vi "Load_vs_Position_Simulation_Model.vi"(0 "Load Setpoint":dbl=20.0 format="%#_13g", 7 "Disturbance":dbl=1.0 format="%#_13g") -> (6 "Simulated Load":dbl, 10 "Simulated Position":dbl)   [LabVIEW 2019]
uses:
  <vilib>/Analysis/1siggen.llb/Ramp Pattern by Samples.vi
  <vilib>/Analysis/NI_AALBase.lvlib
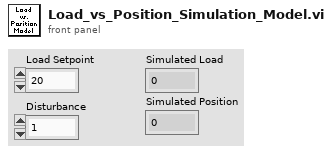
[diagram p1: front panel]
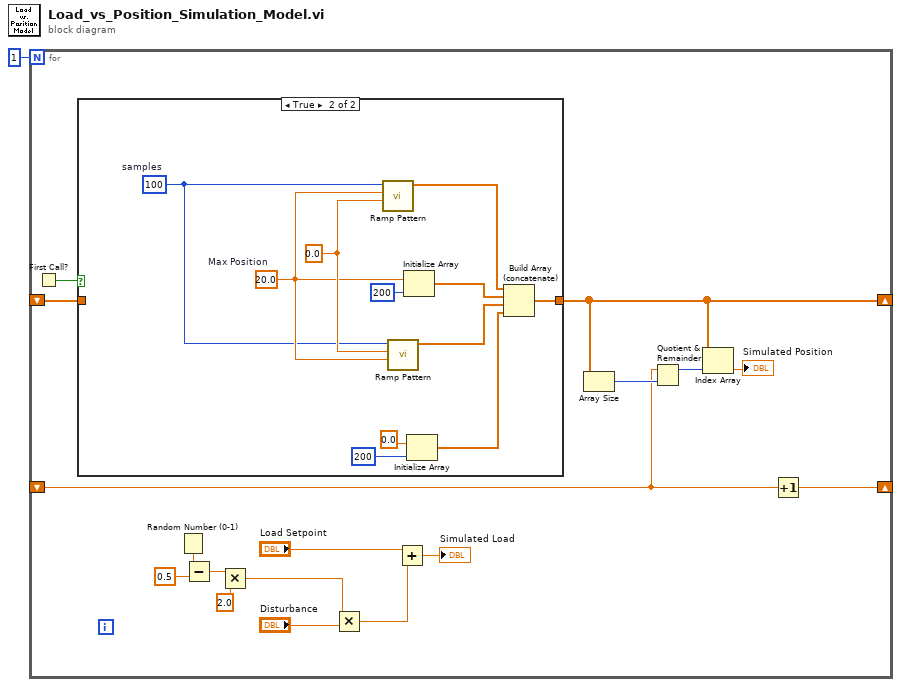
[diagram p0: block diagram]
diagram:
  n1 = for {
    N: 1 -> [_]
    shift-right: [w11] -> _
    shift-left: _ -> [w10]
    shift-right: [w8] -> _
    shift-left: _ -> [w7]
    n2 = First Call?() -> (First Call?: T/F=w9:bool)
    n3 = case shown="True" w9 {
      tunnel: [w19 w30] -> w8
      tunnel: w7 -> [w19 _]
      frame False {
      }
      frame True {
        w21 = 20.0  # Max Position
        w20 = 100  # samples
        w22 = 0.0 ("end")
        n4 = call-poly <vilib>:"Ramp Pattern.vi"("start"=w22, "end"=w21, "samples"=w20) -> ("Ramp Pattern"=w23:dbl[])  [unwired: 7 in, 1 out]
        n5 = call-poly <vilib>:"Ramp Pattern.vi"("start"=w21, "end"=w22, "samples"=w20) -> ("Ramp Pattern"=w25:dbl[])  [unwired: 7 in, 1 out]
        n6 = Initialize Array(w21, 200 ("dimension size")) -> (w26:dbl[])
        n7 = Initialize Array(0.0 ("element"), 200 ("dimension size")) -> (w24:dbl[])
        n8 = Build Array (concatenate)(w23, w26, w25, w24) -> (w30:dbl[])
      }
    }
    n9 = Random Number (0-1)() -> (number: 0 to 1=w6:dbl)
    n10 = Subtract(x=w6, y=0.5) -> (x-y=w4:dbl)
    n11 = Multiply(x=w4, y=2.0) -> (x*y=w2:dbl)
    n12 = Multiply(x=w2, y="Disturbance") -> (x*y=w16:dbl)
    n13 = Add(x="Load Setpoint", y=w16) -> (x+y=→"Simulated Load":dbl)
    n14 = Array Size(array=w8) -> (size(s)=w13:i32)
    n15 = Quotient & Remainder(x=w10, y=w13) -> (x-y*floor(x/y)=w12:i32)  [unwired: 1 out]
    n16 = Index Array(array=w8, index=w12) -> (element=→"Simulated Position":dbl)
    n17 = Increment(x=w10) -> (x+1=w11:dbl)
  }
